vi "DAC Example (A).vi"() -> ()   [LabVIEW 2011]
uses:
  C:/Program Files/Metrohm Autolab/Autolab SDK 1.10/EcoChemie.Autolab.Sdk.dll
  EcoChemie.Autolab.Sdk.dll
panel:
  in  "voltage":dbl
  in  "channel":i32=3 min=0 max=16
  out "error out":errorcluster
  in  "stop":bool
  out "IsConnected":bool
  in  "Hardware Setup File":path
  in  "Embedded Exe File":path
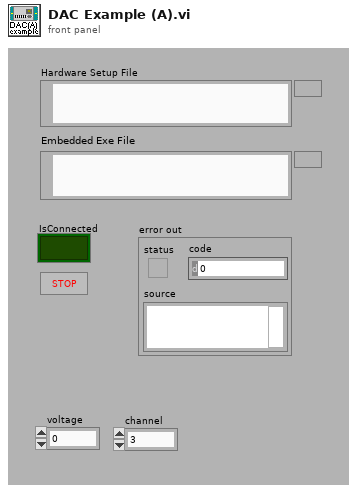
[diagram p1: front panel]
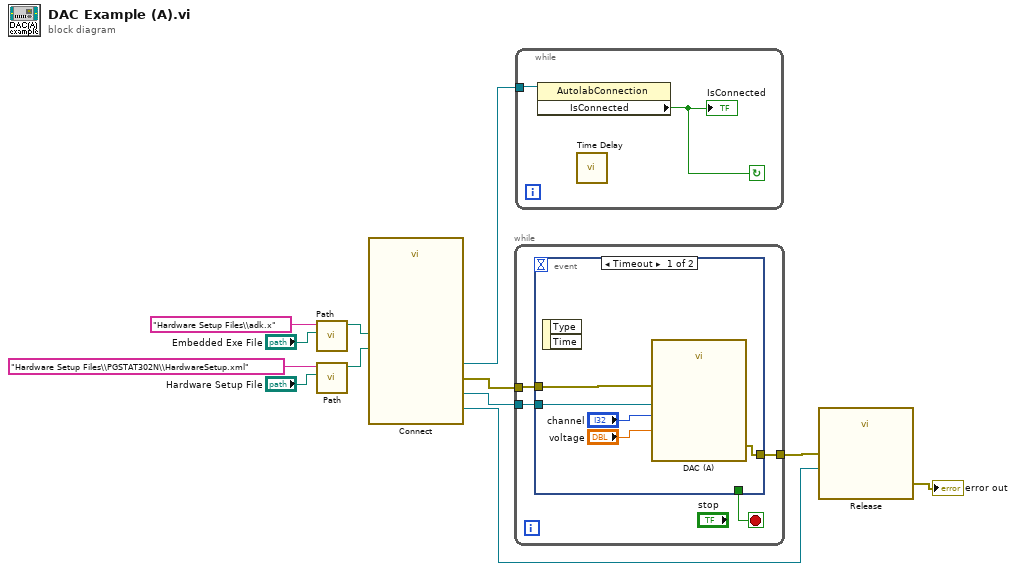
[diagram p0: block diagram]
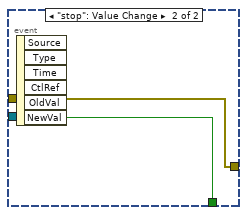
[diagram p2: hidden frame]
diagram:
  n1 = call "Path.vi"("File"="Embedded Exe File", "name or relative path"="Hardware Setup Files\\adk.x") -> ("appended path"=w4:path)  [unwired: 9 in]
  n2 = call "Path.vi"("File"="Hardware Setup File", "name or relative path"="Hardware Setup Files\\PGSTAT302N\\HardwareSetup.xml") -> ("appended path"=w3:path)  [unwired: 9 in]
  n3 = call "Connect.vi"("Embedded Exe File"=w4, "Hardware Setup File"=w3) -> ("Dac"=w8:refnum<k24>, "AutolabConnection"=w10:refnum<k24>, "instrument"=w7:refnum<k24>, "error out"=w9:errorcluster)  [unwired: 6 in, 4 out]
  n4 = while {
    tunnel: w8 -> [w16]
    tunnel: w9 -> [w14]
    tunnel: [w15] -> w11
    stop <- w13 stop-if-true
    n5 = event shown="[0] Timeout" {
      selector: _ -> [_ _]
      dyn-events: _ -> [_ _]
      timeout: _ -> [_ _]
      tunnel: w16 -> [w21 _]
      tunnel: [w18 w22] -> w15
      tunnel: w14 -> [w17 w22]
      tunnel: [_ w23] -> w13
      event Timeout {
        n6 = event-data() -> ()  [unwired: 1 in, 2 out]
        n7 = call "DAC (A).vi"("error in (no error)"=w17, "voltage"="voltage", "channel"="channel", "Dac"=w21) -> ("error out"=w18:errorcluster)  [unwired: 7 in]
      }
      event "stop": Value Change {
        n8 = event-data() -> ("NewVal"=w23:bool)  [unwired: 1 in, 5 out]
      }
    }
  }
  n9 = while {
    tunnel: w10 -> [w25]
    stop <- w24 continue-if-true
    n10 = property class="AutolabConnection"(reference=w25) -> ("IsConnected"=w24:bool)  [unwired: 1 in, 2 out]
    "IsConnected" <- w24
    n11 = call "Time Delay"() -> ()  [unwired: 11 in, 1 out]
  }
  n12 = call "Release.vi"("error in (no error)"=w11, "Instrument"=w7) -> ("error out"=→"error out":errorcluster)  [unwired: 9 in]
